vi "XYZ Stage-Response parser for coordinates.vi"(8 "error in (no error)":errorcluster, 11 "Filtered response string (no CR)":string="111\t333\t444") -> (0 "error out":errorcluster, 1 "Z":sgl, 2 "Y":sgl, 3 "X":sgl)   [LabVIEW 2020]
panel:
  out "before substring 3":string
  out "before substring 2":string
  out "match substring":string
  out "before substring 1":string
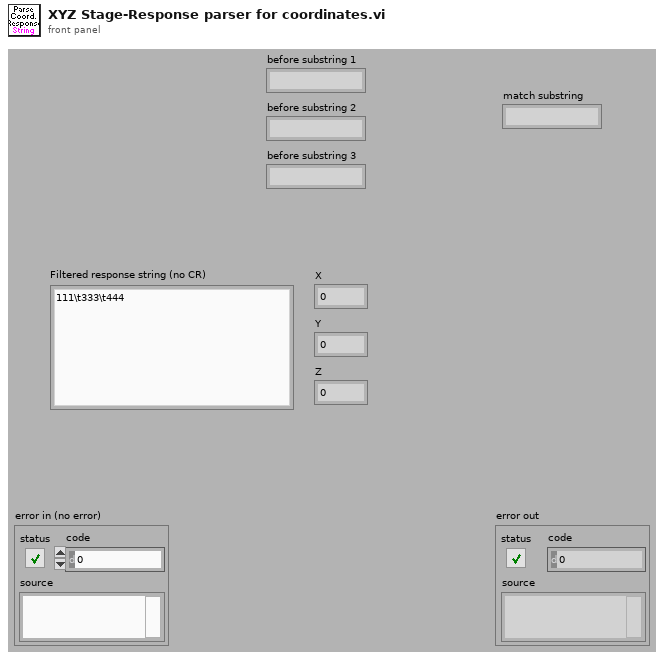
[diagram p1: front panel]
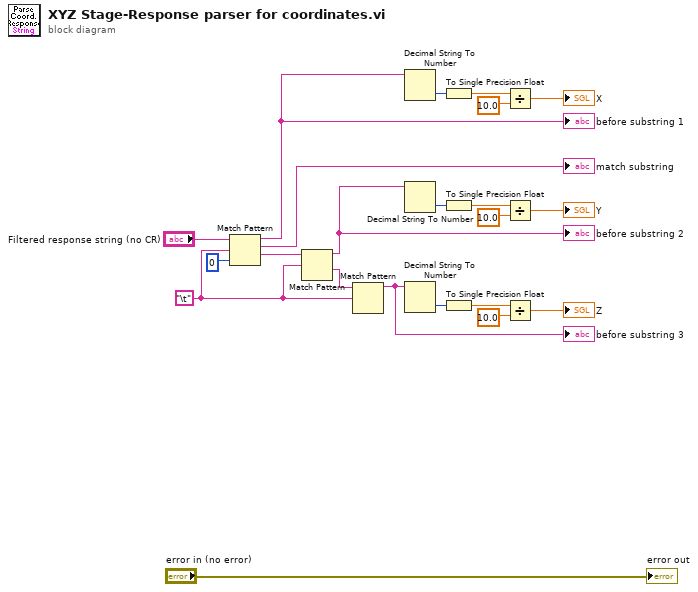
[diagram p0: block diagram]
diagram:
  w18 = "\t"
  n1 = Match Pattern(string="Filtered response string (no CR)", regular expression=w18, offset (0)=0) -> (before substring=w16:string, match substring=→"match substring":string, after substring=w19:string)  [unwired: 1 out]
  "before substring 1" <- w16
  n2 = Match Pattern(string=w19, regular expression=w18) -> (before substring=w15:string, after substring=w17:string)  [unwired: 1 in, 2 out]
  "before substring 2" <- w15
  n3 = Match Pattern(string=w17, regular expression=w18) -> (before substring=w14:string)  [unwired: 1 in, 3 out]
  "before substring 3" <- w14
  n4 = Decimal String To Number(string=w16) -> (number=w13:i32)  [unwired: 2 in, 1 out]
  n5 = Decimal String To Number(string=w15) -> (number=w10:i32)  [unwired: 2 in, 1 out]
  n6 = Decimal String To Number(string=w14) -> (number=w8:i32)  [unwired: 2 in, 1 out]
  n7 = To Single Precision Float(number=w13) -> (single precision float=w2:sgl)
  n8 = To Single Precision Float(number=w10) -> (single precision float=w3:sgl)
  n9 = To Single Precision Float(number=w8) -> (single precision float=w4:sgl)
  n10 = Divide(x=w2, y=sgl 10.0) -> (x/y=→"X":sgl)
  n11 = Divide(x=w3, y=sgl 10.0) -> (x/y=→"Y":sgl)
  n12 = Divide(x=w4, y=sgl 10.0) -> (x/y=→"Z":sgl)
  "error out" <- "error in (no error)"
